vi "Start AuroraTracker.vi"(8 "Error In":errorcluster, 11 "Aurora COM Port":T1=enum."COM4") -> (0 "Error Out":errorcluster)   [LabVIEW 2017]
uses:
  Controls/COM Port.ctl
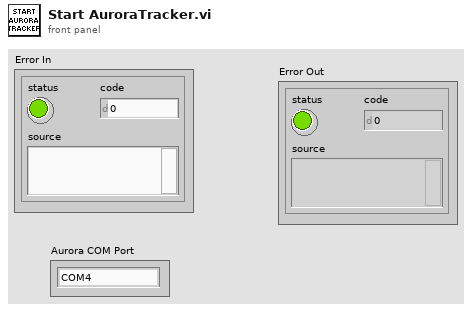
[diagram p1: front panel]
types:
  T1 = typedef "COM Port.ctl" = enum16{"COM1", "COM2", "COM3", "COM4", "COM5", "COM6", "COM7", "COM8", "COM9", "COM10", "COM11", "COM12", "COM13", "COM14", "COM15", "COM16", "COM17", "COM18", "COM19", "COM20"}
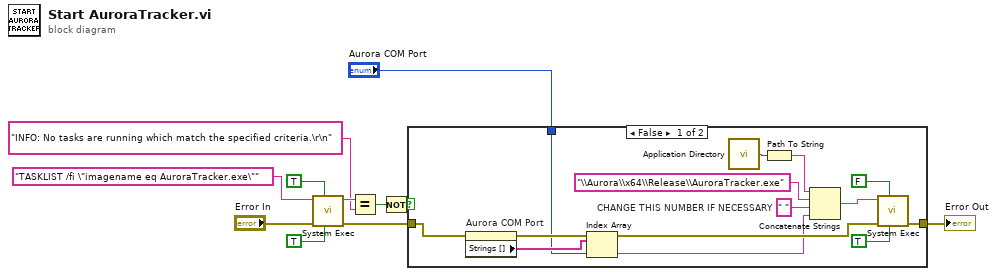
[diagram p0: block diagram]
diagram:
  n1 = call <vilib>:"System Exec.vi"("run minimized? (F)"=TRUE, "wait until completion? (T)"=TRUE, "error in (no error)"="Error In", "command line"="TASKLIST /fi \"imagename eq AuroraTracker.exe\"" ("String")) -> ("error out"=w3:errorcluster, "standard output"=w10:string)  [unwired: 4 in, 2 out]
  n2 = Equal?(x=w10, y="INFO: No tasks are running which match the specified criteria.\r\n") -> (x = y?=w9:bool)
  n3 = Not(x=w9) -> (.not. x?=w5:bool)
  n4 = case shown="False" w5 {
    tunnel: w3 -> [w16 w25]
    tunnel: [w22 w25] -> w4
    tunnel: "Aurora COM Port" -> [w13 _]
    frame False {
      w19 = " "  # CHANGE THIS NUMBER IF NECESSARY
      n5 = property on="Aurora COM Port" class="Enum (strict)"(error in=w16) -> (error out=w15:errorcluster, "Strings []"=w14:string[])  [unwired: 1 in, 1 out]
      n6 = Index Array(array=w14, index=w13) -> (element=w12:string)
      n7 = call <vilib>:"Application Directory.vi"() -> ("Application Directory"=w17:path)
      n8 = Path To String(path=w17) -> (string=w21:string)
      n9 = Concatenate Strings(w21, "\\Aurora\\x64\\Release\\AuroraTracker.exe" ("name or relative path"), w19, w12) -> (w20:string)
      n10 = call <vilib>:"System Exec.vi"("run minimized? (F)"=TRUE, "wait until completion? (T)"=FALSE, "error in (no error)"=w15, "command line"=w20) -> ("error out"=w22:errorcluster)  [unwired: 4 in, 3 out]
    }
    frame True {
    }
  }
  "Error Out" <- w4
